vi "turretPitchLogical.vi"(0 "softstop":dbl, 1 "tolerance":dbl, 2 "evalPeriod":dbl, 4 "PID gains":T1={"proportional gain (Kc)"=1.0, "integral time (Ti, min)"=0.01, "derivative time (Td, min)"=0.0} {"derivative time (Td, min)" format="%.3f"; "integral time (Ti, min)" format="%.3f"; "proportional gain (Kc)" format="%.3f"}, 5 "desiredAngle":dbl format="%.2f", 6 "output range":cluster{"output high":dbl, "output low":dbl}={"output high"=100.0, "output low"=-100.0} {"output low" format="%.2f"; "output high" format="%.2f"}, 7 "range":cluster{"high":dbl, "low":dbl}, 8 "currentAngle":dbl format="%.2f", 9 "servoPitchDevRef":T2={"DeviceStatus"={"status"=FALSE, "code"=0, "source"=""}, "PWM Channel"=enum."Invalid", "DeadBand"={"Name"="", "maxPositivePwm"=0, "minPositivePwm"=0, "centerPwm"=0, "maxNegativePwm"=0, "minNegativePwm"=0, "angularRange"=0}}) -> (3 "done":bool)   [LabVIEW 2016]
uses:
  <vilib>/Rock Robotics/WPI/PWM/Servo/WPI_ServoDeviceRef.ctl
  <vilib>/Rock Robotics/SystemInterfaces/DIO/FPGA_DIOPWMChannel.ctl
  <vilib>/Rock Robotics/WPI/PWM/WPI_PWMDeadband.ctl
  <vilib>/addons/control/pid/pid.llb/PID (DBL).vi
  <vilib>/addons/control/pid/NI_PID_pid.lvlib
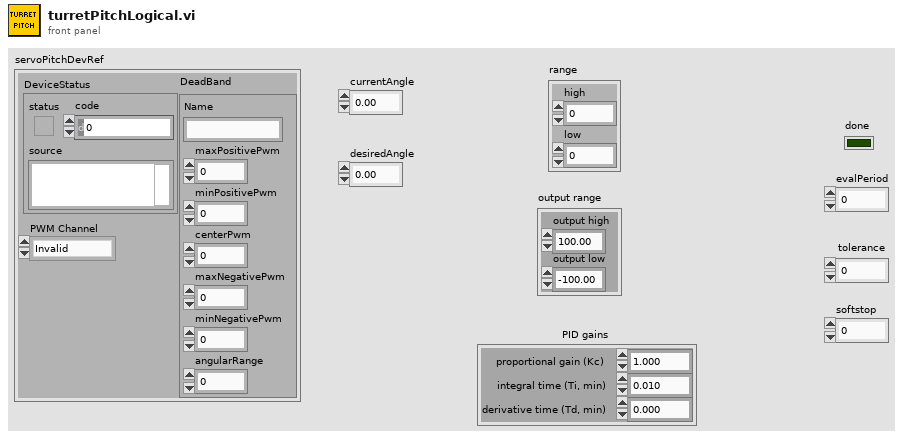
[diagram p1: front panel]
types:
  T1 = cluster{"proportional gain (Kc)":dbl, "integral time (Ti, min)":dbl, "derivative time (Td, min)":dbl}
  T2 = typedef "WPI_ServoDeviceRef.ctl" = cluster{"DeviceStatus":errorcluster, "PWM Channel":T3, "DeadBand":T4}
  T3 = typedef "FPGA_DIOPWMChannel.ctl" = enum8{"PWM 0", "PWM 1", "PWM 2", "PWM 3", "PWM 4", "PWM 5", "PWM 6", "PWM 7", "PWM 8", "PWM 9", "PWM MXP 0", "PWM MXP 1", "PWM MXP 2", "PWM MXP 3", "PWM MXP 4", "PWM MXP 5", "PWM MXP 6", "PWM MXP 7", "PWM MXP 8", "PWM MXP 9", "Invalid"}
  T4 = typedef "WPI_PWMDeadband.ctl" = cluster{"Name":string, "maxPositivePwm":i32, "minPositivePwm":i32, "centerPwm":i32, "maxNegativePwm":i32, "minNegativePwm":i32, "angularRange":u16}
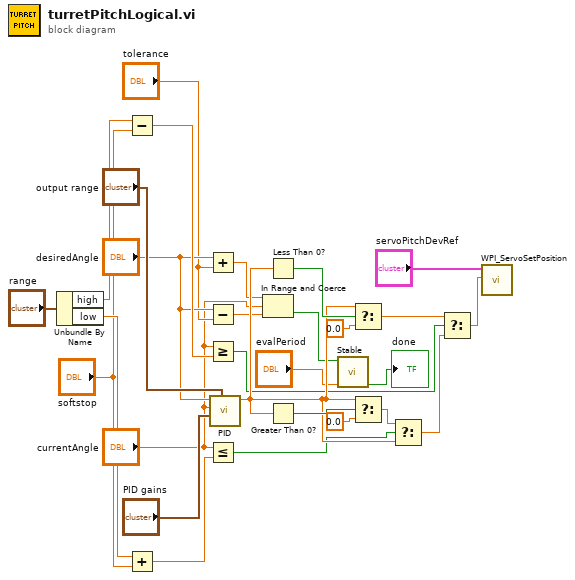
[diagram p0: block diagram]
diagram:
  n1 = Unbundle By Name("range") -> ("high"=w18:dbl, "low"=w17:dbl)
  n2 = Subtract(x=w18, y="softstop") -> (x-y=w12:dbl)
  n3 = Add(x=w17, y="softstop") -> (x+y=w10:dbl)
  n4 = Add(x="desiredAngle", y="tolerance") -> (x+y=w6:dbl)
  n5 = Subtract(x="desiredAngle", y="tolerance") -> (x-y=w5:dbl)
  n6 = Greater Or Equal?(x="currentAngle", y=w12) -> (x >= y?=w11:bool)
  n7 = Less Or Equal?(x="currentAngle", y=w10) -> (x <= y?=w9:bool)
  n8 = call-poly <vilib>:"PID.vi"("output range"="output range", "PID gains"="PID gains", "process variable"="currentAngle", "setpoint"="desiredAngle") -> ("output"=w13:dbl)  [unwired: 6 in, 1 out]
  n9 = In Range and Coerce(upper limit=w6, x="currentAngle", lower limit=w5) -> (In Range?=w4:bool)  [unwired: 1 out]
  n10 = Less Than 0?(x=w13) -> (x < 0?=w15:bool)
  n11 = Greater Than 0?(x=w13) -> (x > 0?=w14:bool)
  n12 = call <userlib>:"Stable.vi"("Eval Period (sec)"="evalPeriod", "Signal Input"=w4) -> ("Stable"=→"done":bool)  [unwired: 9 in]
  n13 = Select(t=w13, s=w15, f=0.0) -> (s? t:f=w22:dbl)
  n14 = Select(t=w13, s=w14, f=0.0) -> (s? t:f=w21:dbl)
  n15 = Select(t=w21, s=w9, f=w13) -> (s? t:f=w23:dbl)
  n16 = Select(t=w22, s=w11, f=w23) -> (s? t:f=w24:dbl)
  n17 = call <vilib>:"WPI_ServoSetPosition.vi"("Position"=w24, "ServoDeviceRef"="servoPitchDevRef") -> ()  [unwired: 8 in, 2 out]
